vi "AMZ_S3_HMAC-SHA-1.vi"(1 "Key":string, 2 "Message":string) -> (0 "Digest":string)   [LabVIEW 2015, in "LV Interface for Amazon S3.lvlib"]
doc: "Signs the Message with Key using HMAC SHA-1 algorithm."
uses:
  LV Interface for Amazon S3.lvlib
  SHA-1/SHA-1 Core.vi
  SHA-1/SHA-1 Digest.vi
  SHA-1/SHA-1 Pad.vi
  SHA-1/SHA-1.lvlib
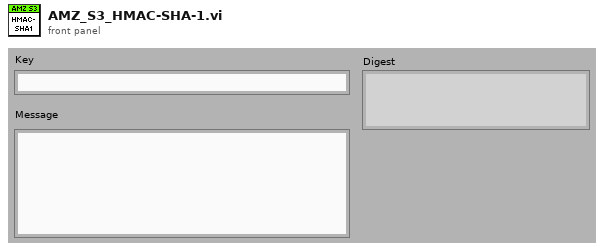
[diagram p1: front panel]
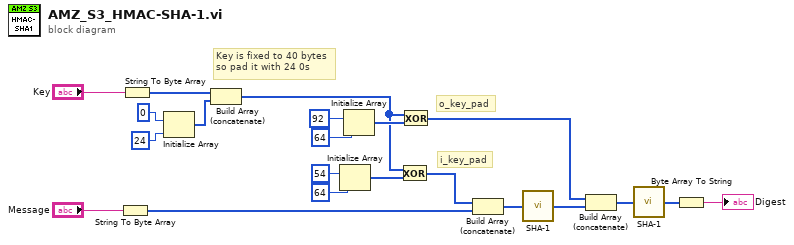
[diagram p0: block diagram]
diagram:
  # "Key is fixed to 40 bytes\nso pad it with 24 0s"
  # "i_key_pad"
  # "o_key_pad"
  n1 = String To Byte Array(string="Message") -> (unsigned byte array=w7:u8[])
  n2 = String To Byte Array(string="Key") -> (unsigned byte array=w19:u8[])
  n3 = Initialize Array(u8 0, 24 ("dimension size")) -> (w18:u8[])
  n4 = Build Array (concatenate)(w19, w18) -> (w10:u8[])
  n5 = Initialize Array(u8 54, 64 ("dimension size")) -> (w11:u8[])
  n6 = Initialize Array(u8 92, 64 ("dimension size")) -> (w14:u8[])
  n7 = Exclusive Or(1:w11, 2:w10) -> (0:w8:u8[])
  n8 = Exclusive Or(1:w14, 2:w10) -> (0:w6:u8[])
  n9 = Build Array (concatenate)(w8, w7) -> (w4:u8[])
  n10 = call "SHA-1.vi"("Data"=w4) -> ("message-digest"=w3:u8[])
  n11 = Build Array (concatenate)(w6, w3) -> (w2:u8[])
  n12 = call "SHA-1.vi"("Data"=w2) -> ("message-digest"=w1:u8[])
  n13 = Byte Array To String(unsigned byte array=w1) -> (string=→"Digest":string)
